vi "Disabled.vi"(7 "Robot Mode":T2, 10 "Match Info":T1={"Autonomous Elapsed Seconds"=0.0, "TeleOp Elapsed Seconds"=0.0, "Disabled Elapsed Seconds"=0.0, "Visited Autonomous"=FALSE, "Visited TeleOp"=FALSE, "Visited Disabled"=FALSE, "Autonomous Settings"={"Autonomous Style"=enum."Independent", "VI Refnum"=refnum}}, 11 "Call Context":T3) -> ()   [LabVIEW 2011]
doc: "This VI is called each time a disabled packet is received from the DS. It is often used to prepare for the next robot mode, to calibrate sensors, etc."
uses:
  <vilib>/Rock Robotics/WPI/DriverStation/WPI_DriverStationDerivedRobotMode.ctl
  <vilib>/Rock Robotics/WPI/DriverStation/WPI_DriverStationRobotMode.ctl
  <vilib>/Rock Robotics/WPI/DriverStation/WPI_DriverStationMatch Info.ctl
  Robot Global Data.vi
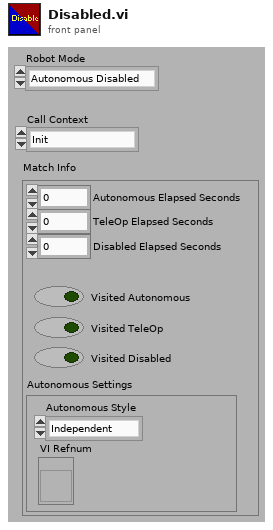
[diagram p1: front panel]
types:
  T1 = typedef "WPI_DriverStationMatch Info.ctl" = cluster{"Autonomous Elapsed Seconds":dbl, "TeleOp Elapsed Seconds":dbl, "Disabled Elapsed Seconds":dbl, "Visited Autonomous":bool, "Visited TeleOp":bool, "Visited Disabled":bool, "Autonomous Settings":cluster{"Autonomous Style":enum16{"Iterative", "Independent"}, "VI Refnum":refnum<vi>}}
  T2 = typedef "WPI_DriverStationRobotMode.ctl" = enum16{"Autonomous Disabled", "Autonomous Enabled", "Teleop Disabled", "Teleop Enabled", "Timeout", "Finish"}
  T3 = typedef "WPI_DriverStationDerivedRobotMode.ctl" = enum16{"Init", "Execute", "Stop"}
  T4 = typedef "WPI_MotorControlDeviceRef.ctl" = cluster{"DeviceStatus":errorcluster, "Type":enum16{"PWM", "CAN"}, "PWM":cluster{"Digital Module":T5, "PWM Channel":T6, "DeadBand":T7}, "CAN":cluster{"Device Number":u8, "Control Mode":T8, "Semaphore":T9, "Max Vout":dbl}, "Invert":bool, "TransformRef":T10, "InvTransformRef":T10}
  T5 = typedef "FPGA_TypedefDigitalModule.ctl" = enum16{"Digital Module 1", "Digital Module 2"}
  T6 = typedef "FPGA_DIOPWMChannel.ctl" = enum8{"PWM 1", "PWM 2", "PWM 3", "PWM 4", "PWM 5", "PWM 6", "PWM 7", "PWM 8", "PWM 9", "PWM 10", "Invalid"}
  T7 = typedef "WPI_PWMDeadband.ctl" = cluster{"Name":string, "maxPositivePwm":i32, "minPositivePwm":i32, "centerPwm":i32, "maxNegativePwm":i32, "minNegativePwm":i32, "angularRange":u16}
  T8 = typedef "WPI_CANJaguar_ControlMode.ctl" = enum8{"Percent VBus", "Current", "Speed", "Position", "Voltage"}
  T9 = typedef "Semaphore RefNum" = refnum<k1>
  T10 = typedef "WPI_PWMTransform_ConPane.ctl" = refnum<vi>
  T11 = typedef "WPI_JoystickDevRef.ctl" = cluster{"Device":T12}
  T12 = typedef "WPI_JoystickDeviceEnum.ctl" = enum16{"USB 1", "USB 2", "USB 3", "USB 4", "Kinect 1", "Kinect 2"}
  T13 = typedef "WPI_JoystickButtonState.ctl" = cluster{"Button 1":bool, "Button 2":bool, "Button 3":bool, "Button 4":bool, "Button 5":bool, "Button 6":bool, "Button 7":bool, "Button 8":bool, "Button 9":bool, "Button 10":bool, "Button 11":bool, "Button 12":bool}
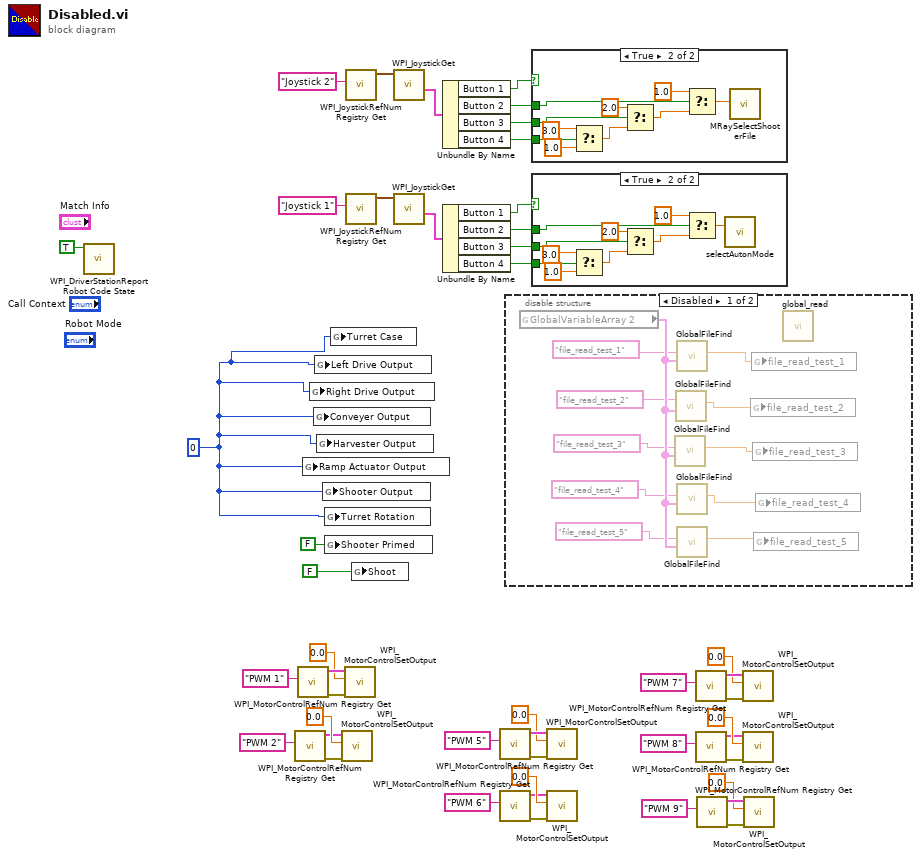
[diagram p0: block diagram]
diagram:
  w15 = 0
  n1 = call <vilib>:"WPI_DriverStationReport Robot Code State.vi"("Disabled"=TRUE ("Autonomous")) -> ()  [unwired: 10 in, 1 out]
  n2 = call <vilib>:"WPI_MotorControlRefNum Registry Get.vi"("refnum name"="PWM 2") -> ("error out"=w39:errorcluster, "MotorControlDevRef"=w38:T4)  [unwired: 9 in]
  n3 = call <vilib>:"WPI_MotorControlRefNum Registry Get.vi"("refnum name"="PWM 1") -> ("error out"=w44:errorcluster, "MotorControlDevRef"=w45:T4)  [unwired: 9 in]
  n4 = global write "Robot Global Data.vi" "Ramp Actuator Output"(w15) -> ()
  n5 = global write "Robot Global Data.vi" "Right Drive Output"(w15) -> ()
  n6 = global write "Robot Global Data.vi" "Conveyer Output"(w15) -> ()
  n7 = global write "Robot Global Data.vi" "Left Drive Output"(w15) -> ()
  n8 = global write "Robot Global Data.vi" "Harvester Output"(w15) -> ()
  n9 = global write "Robot Global Data.vi" "Shooter Output"(w15) -> ()
  n10 = global write "Robot Global Data.vi" "Turret Rotation"(w15) -> ()
  n11 = global write "Robot Global Data.vi" "Shooter Primed"(FALSE ("Shooter Primed")) -> ()
  n12 = global write "Robot Global Data.vi" "Turret Case"(w15) -> ()
  n13 = call <vilib>:"WPI_MotorControlSetOutput.vi"("error in (no error)"=w39, "Output"=0.0, "MotorControlDevRef"=w38) -> ()  [unwired: 7 in, 2 out]
  n14 = call <vilib>:"WPI_MotorControlSetOutput.vi"("error in (no error)"=w44, "Output"=0.0, "MotorControlDevRef"=w45) -> ()  [unwired: 7 in, 2 out]
  n15 = call <vilib>:"WPI_JoystickRefNum Registry Get.vi"("refnum name"="Joystick 2") -> ("JoystickDevRef"=w2:T11)  [unwired: 9 in, 1 out]
  n16 = call <vilib>:"WPI_JoystickRefNum Registry Get.vi"("refnum name"="Joystick 1") -> ("JoystickDevRef"=w13:T11)  [unwired: 9 in, 1 out]
  n17 = global write "Robot Global Data.vi" "Shoot"(FALSE ("Shooter Primed")) -> ()
  n18 = call <vilib>:"WPI_JoystickGet.vi"("JoystickDevRef"=w2) -> ("Buttons"=w3:T13)  [unwired: 4 in, 2 out]
  n19 = call <vilib>:"WPI_JoystickGet.vi"("JoystickDevRef"=w13) -> ("Buttons"=w12:T13)  [unwired: 4 in, 2 out]
  n20 = Unbundle By Name(w3) -> ("Button 1"=w4:bool, "Button 2"=w5:bool, "Button 3"=w6:bool, "Button 4"=w7:bool)
  n21 = Unbundle By Name(w12) -> ("Button 1"=w11:bool, "Button 2"=w10:bool, "Button 3"=w9:bool, "Button 4"=w8:bool)
  n22 = call <vilib>:"WPI_MotorControlRefNum Registry Get.vi"("refnum name"="PWM 5") -> ("error out"=w36:errorcluster, "MotorControlDevRef"=w37:T4)  [unwired: 9 in]
  n23 = call <vilib>:"WPI_MotorControlRefNum Registry Get.vi"("refnum name"="PWM 6") -> ("error out"=w31:errorcluster, "MotorControlDevRef"=w30:T4)  [unwired: 9 in]
  n24 = disable-structure shown="Disabled" {
    frame Disabled {
      n25 = global read "Robot Global Data.vi" "GlobalVariableArray 2"() -> (w57:cluster{"name":string, "va;":dbl}[])
      n26 = call "GlobalFileFind.vi"("GlobalVariableArray 2"=w57, "VariableNameLookup"="file_read_test_3") -> ("VariableValueOut"=w48:dbl)  [unwired: 9 in]
      n27 = call "GlobalFileFind.vi"("GlobalVariableArray 2"=w57, "VariableNameLookup"="file_read_test_2") -> ("VariableValueOut"=w47:dbl)  [unwired: 9 in]
      n28 = call "GlobalFileFind.vi"("GlobalVariableArray 2"=w57, "VariableNameLookup"="file_read_test_1") -> ("VariableValueOut"=w51:dbl)  [unwired: 9 in]
      n29 = call "GlobalFileFind.vi"("GlobalVariableArray 2"=w57, "VariableNameLookup"="file_read_test_4") -> ("VariableValueOut"=w49:dbl)  [unwired: 9 in]
      n30 = call "GlobalFileFind.vi"("GlobalVariableArray 2"=w57, "VariableNameLookup"="file_read_test_5") -> ("VariableValueOut"=w50:dbl)  [unwired: 9 in]
      n31 = global write "Robot Global Data.vi" "file_read_test_2"(w47) -> ()
      n32 = global write "Robot Global Data.vi" "file_read_test_1"(w51) -> ()
      n33 = global write "Robot Global Data.vi" "file_read_test_3"(w48) -> ()
      n34 = global write "Robot Global Data.vi" "file_read_test_5"(w50) -> ()
      n35 = global write "Robot Global Data.vi" "file_read_test_4"(w49) -> ()
      n36 = call "global_read.vi"() -> ()  [unwired: 12 in]
    }
    frame Enabled {
    }
  }
  n37 = case shown="True" w4 {
    tunnel: w5 -> [_ w64]
    tunnel: w6 -> [_ w62]
    tunnel: w7 -> [_ w67]
    frame False {
    }
    frame True {
      n38 = Select(t=3.0, s=w67, f=1.0) -> (s? t:f=w60:dbl)
      n39 = Select(t=2.0, s=w62, f=w60) -> (s? t:f=w59:dbl)
      n40 = Select(t=1.0, s=w64, f=w59) -> (s? t:f=w58:dbl)
      n41 = call "MRaySelectShooterFile.vi"("Shooter File"=w58) -> ()  [unwired: 11 in]
    }
  }
  n42 = case shown="True" w11 {
    tunnel: w10 -> [_ w74]
    tunnel: w9 -> [_ w72]
    tunnel: w8 -> [_ w77]
    frame False {
    }
    frame True {
      n43 = Select(t=3.0, s=w77, f=1.0) -> (s? t:f=w70:dbl)
      n44 = Select(t=2.0, s=w72, f=w70) -> (s? t:f=w69:dbl)
      n45 = Select(t=1.0, s=w74, f=w69) -> (s? t:f=w68:dbl)
      n46 = call "selectAutonMode.vi"("Auton File"=w68) -> ()  [unwired: 2 in]
    }
  }
  n47 = call <vilib>:"WPI_MotorControlSetOutput.vi"("error in (no error)"=w36, "Output"=0.0, "MotorControlDevRef"=w37) -> ()  [unwired: 7 in, 2 out]
  n48 = call <vilib>:"WPI_MotorControlSetOutput.vi"("error in (no error)"=w31, "Output"=0.0, "MotorControlDevRef"=w30) -> ()  [unwired: 7 in, 2 out]
  n49 = call <vilib>:"WPI_MotorControlRefNum Registry Get.vi"("refnum name"="PWM 7") -> ("error out"=w28:errorcluster, "MotorControlDevRef"=w29:T4)  [unwired: 9 in]
  n50 = call <vilib>:"WPI_MotorControlRefNum Registry Get.vi"("refnum name"="PWM 8") -> ("error out"=w23:errorcluster, "MotorControlDevRef"=w22:T4)  [unwired: 9 in]
  n51 = call <vilib>:"WPI_MotorControlRefNum Registry Get.vi"("refnum name"="PWM 9") -> ("error out"=w20:errorcluster, "MotorControlDevRef"=w21:T4)  [unwired: 9 in]
  n52 = call <vilib>:"WPI_MotorControlSetOutput.vi"("error in (no error)"=w28, "Output"=0.0, "MotorControlDevRef"=w29) -> ()  [unwired: 7 in, 2 out]
  n53 = call <vilib>:"WPI_MotorControlSetOutput.vi"("error in (no error)"=w23, "Output"=0.0, "MotorControlDevRef"=w22) -> ()  [unwired: 7 in, 2 out]
  n54 = call <vilib>:"WPI_MotorControlSetOutput.vi"("error in (no error)"=w20, "Output"=0.0, "MotorControlDevRef"=w21) -> ()  [unwired: 7 in, 2 out]
